vi "DELETE Samples Per Sweep.vi"   [LabVIEW 2013]
uses:
  Action.ctl
  Calibration Input FGV Selector.ctl
types:
  T1 = typedef "Calibration Input FGV Selector.ctl" = enum16{"Samples/Sweep", "Num Sweeps", "Sample Rate"}
  T2 = typedef "Action.ctl" = enum16{"GET", "PUT", "DELETE"}
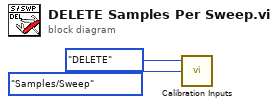
[diagram p0: block diagram]
diagram:
  n1 = call "Calibration Inputs.vi"("Calibration Input FGV Selector"=Calibration_Input_FGV_Selector."Samples/Sweep", "Verb"=Action."DELETE") -> ()  [unwired: 1 in, 1 out]
